vi "Get FPGA Name.vi"(8 "error in (no error)":errorcluster, 11 "Schedule Cell in":refnum<class "Schedule Cell.lvclass">) -> (0 "error out":errorcluster, 2 "FPGA Name":string, 3 "Schedule Cell out":refnum<class "Schedule Cell.lvclass">)   [LabVIEW 2020, in "Run Utilities.lvlib" / "Schedule Cell.lvclass"]
uses:
  Schedule Cell.lvclass
  Run Instance/Run Instance.lvclass
  Schedule Cell.lvclass/Schedule Cell.ctl
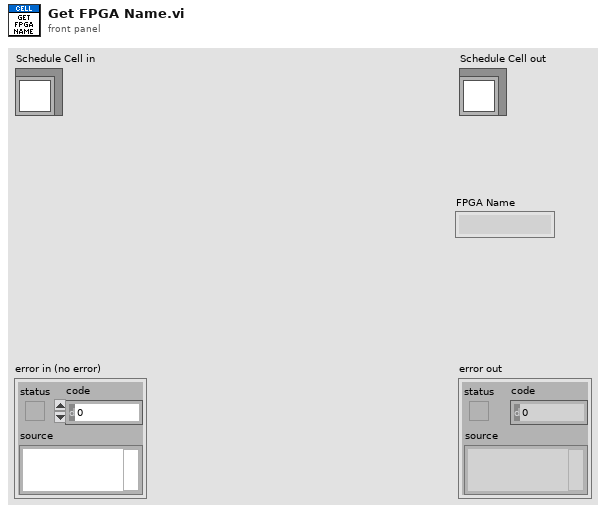
[diagram p1: front panel]
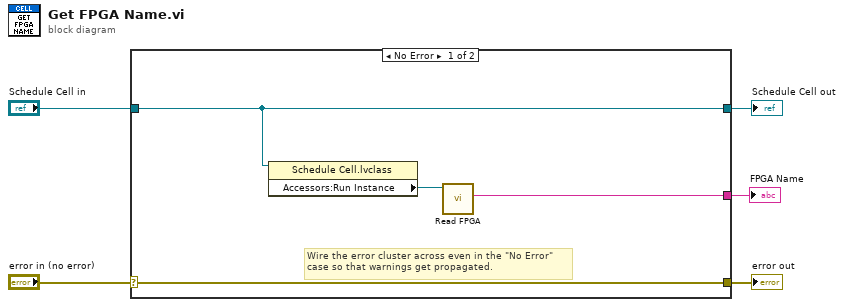
[diagram p0: block diagram]
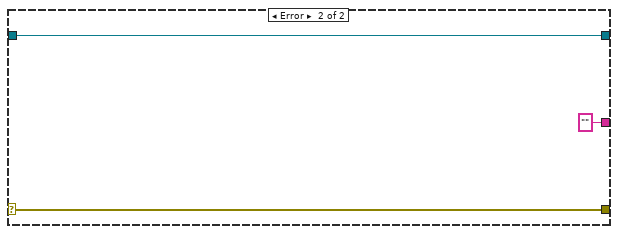
[diagram p2: hidden frame]
diagram:
  n1 = case shown="No Error" "error in (no error)" {
    selector: "error in (no error)" -> [w9 w12]
    tunnel: [w9 w12] -> w4
    tunnel: [w7 w11] -> w2
    tunnel: "Schedule Cell in" -> [w7 w11]
    tunnel: [w6 ""] -> w1
    frame No Error {
      # "Wire the error cluster across even in the \"No Error\"\ncase so that warnings get propagated."
      n2 = property class="Schedule Cell.lvclass"(reference=w7) -> ("Accessors:Run Instance"=w8:refnum<class "Run Instance.lvclass">)  [unwired: 1 in, 2 out]
      n3 = call-dynamic "Read FPGA.vi"("Run Instance in"=w8) -> ("FPGA Name"=w6:string)  [unwired: 8 in, 2 out]
    }
    frame Error {
    }
  }
  "error out" <- w4
  "Schedule Cell out" <- w2
  "FPGA Name" <- w1
